vi "Controller Analog to Joystick Analog.vi"(1 "Controller Value":i32) -> (0 "Joystick Value":dbl)   [LabVIEW 2018]
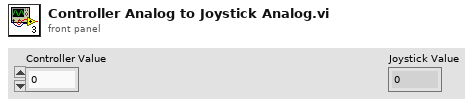
[diagram p1: front panel]
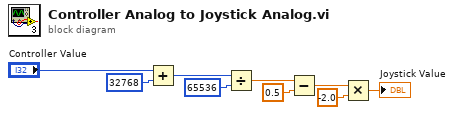
[diagram p0: block diagram]
diagram:
  n1 = Add(x="Controller Value", y=32768) -> (x+y=w7:i32)
  n2 = Divide(x=w7, y=65536) -> (x/y=w5:dbl)
  n3 = Subtract(x=w5, y=0.5) -> (x-y=w3:dbl)
  n4 = Multiply(x=w3, y=-2.0) -> (x*y=→"Joystick Value":dbl)
